vi "NavbalLabVIEW(15-5-21).vi"() -> ()   [LabVIEW 2010]
uses:
  <vilib>/Analysis/Matrix/Datatypes/RealMatrix.ctl
  <vilib>/Utility/NIReport.llb/HTML Report Image Alignment.ctl
  <vilib>/Utility/NIReport.llb/NI_report.lvclass
  <vilib>/Analysis/Matrix/Datatypes/ComplexMatrix.ctl
  <userlib>/Circular Buffer/Controls/Circular Buffer Operations.ctl
  <vilib>/addons/_office/_exclsub.llb/font.ctl
  <vilib>/addons/_office/excel.llb/Excel Get Data ([str]).vi
  <vilib>/addons/_office/excel.llb/Excel Get Data ([i32]).vi
  <vilib>/Analysis/Matrix/Numeric/Multiply/Multiply - R,RM.vi
  <vilib>/Analysis/Matrix/Numeric/Complex/Polar To Complex - RM,RM.vi
  <vilib>/Analysis/Matrix/Numeric/Conversions/Matrix To Array - RM.vi
  <vilib>/Analysis/Matrix/Numeric/Conversions/Array To Matrix - CA2.vi
  <vilib>/Analysis/Matrix/Numeric/Multiply/Multiply - RM,R.vi
  <vilib>/Analysis/baseanly.llb/Complex A x B.vi
  <vilib>/Analysis/Matrix/Numeric/Add/Add - CM,CM.vi
  <vilib>/Analysis/Matrix/Numeric/Complex/Complex To Polar - CM.vi
  <vilib>/Analysis/Matrix/Numeric/Subtract/Subtract - RM,RM.vi
  <vilib>/addons/_office/excel.llb/Excel Get Data ([dbl]).vi
  <userlib>/Circular Buffer/Instance VIs/Circular Buffer(2D Wfm with Attributes).vi
  <vilib>/addons/_office/excel.llb/Excel Easy Table (str).vi
  <vilib>/addons/_NISVFA/_Shared subVIs/Common/SVL Set dB Reference (N Ch - 1 Ref).vi
  <vilib>/measure/matone.llb/Extract Single Tone Information N Chan.vi
  <vilib>/Analysis/NI_AALPro.lvlib
  <vilib>/Utility/NIReport.llb/NI_ReportGenerationCore.lvlib
  <vilib>/Analysis/Matrix/NI_Matrix.lvlib
  <userlib>/Circular Buffer/Circular Buffer.lvlib
  <vilib>/measure/NI_MAPro.lvlib
  <vilib>/Utility/NIReport.llb/Excel/NI_Excel.lvclass
  <vilib>/addons/_office/NI_ReportGenerationToolkit.lvlib
  <vilib>/ptbypt/NI_PtbyPt.lvlib
  <vilib>/Analysis/NI_AALBase.lvlib
panel:
  in  "Print Button":bool caption="Blank Button"
  in  "Averaging":bool
  in  "Number of Averages":i32=100
  in  "Tab 2":T1(tab)
  in  "Save BG":bool
  out "XY Graph":cluster{"y vector":sgl[], dbl[]}[](graph)
  out "Port 60":dbl[](array[numeric])
  out "Stbd 60":dbl[](array[numeric])
  out "Corners 60":dbl[](array[numeric])
  out "Corners 120":dbl[](array[numeric])
  out "Stbd 120":dbl[](array[numeric])
  out "Port 120":dbl[](array[numeric])
  out "Sensor Name":string
  out "AdB Starboard":cluster{"x0":dbl, "dx":dbl, dbl[][]}(graph)={"x0"=0.0, "dx"=0.25, []}
  out "Accelerometer Signals Stbd":dynamicdata(graph) caption="Signal Out"
  out "Tach Signal Stbd":dynamicdata(graph) caption="Signal Out"
  out "AdB Port":cluster{"x0":dbl, "dx":dbl, dbl[][]}(graph)={"x0"=0.0, "dx"=0.25, []}
  out "Accelerometer Signals Port":dynamicdata(graph) caption="Signal Out"
  out "Tach Signal Port":dynamicdata(graph) caption="Signal Out"
  out "AdB Corners":cluster{"x0":dbl, "dx":dbl, dbl[][]}(graph)={"x0"=0.0, "dx"=0.25, []}
  out "Accelerometer Signals Corners":dynamicdata(graph) caption="Signal Out"
  in  "MagPhase":i32[](listbox)
  out "Spectrum (AdB)":cluster{"x0":dbl, "dx":dbl, dbl[][]}(graph)
  in  "Save Vibration Survey":bool
  in  "Vibration Survey Name":string
  out "Default Stbd Graph":dynamicdata(graph)
  in  "Enter into log":bool
  in  "Log Input":string
  out "Frequency (RPM) 1":i32=3573 caption="RPM"
  out "Frequency (Hz) 1":dbl=59.548178197923264 caption="Hz" format="%0.2f"
  out "Frequency (RPM) 2":i32=3621 caption="RPM"
  out "Frequency (Hz) 2":dbl=60.35080413674587 caption="Hz" format="%0.2f"
  in  "DAQ Start":bool
  in  "stop 4":bool
  in  "Tab 1":T2(tab)
  in  "Divisions in\nEach Plane S":T3=[[24.0], [24.0], [16.0], [16.0]]
  out "With/Against\nRotation S":string[][](array[string])
  in  "Load File":bool
  in  "Printer Name":string="HP LaserJet Professional P1102w"
  in  "Boat File":path
  in  "Frequency Resolution":u16(ring) items=["0.25 Hz", "0.5 Hz", "1 Hz", "5 Hz", "10 Hz"]
  in  "Frequency Upper Limit":u16(ring)=2 items=["200 Hz", "400 Hz", "800 Hz", "1600 Hz", "3200 Hz", "6400", "12.8 kHz"]
  in  "Ship Class":T4(radio)
  out "Number of Samples":i32
  out "Sample Frequency (Hz)":i32
  out "Sensor Info":string[][](array[string])
  out "sensor end line":cluster{"row":i32, i32}
  out "# Accel Channels":i32
  out "#Corner Accels":i32
  out "#Stbd Accels":i32
  out "#Port Accels":i32
  out "With/Against\nRotation P":string[][](array[string])
  in  "Divisions in\nEach Plane P":T3=[[24.0], [24.0], [16.0], [16.0]]
  in  "Calib Avg":bool
  in  "Accel Calib Start":bool
  out "mV/in/s":dbl
  out "Volts":dbl
  in  "Calibration Channel List":i32(listbox)
  out "FFT mV/in/s":cluster{"x0":dbl, "dx":dbl, "magnitude":dbl[]}[](graph)
  out "Volts Graph":dynamicdata(graph)=[{"t0"=timestamp(3478348950.00005 s since 1904-01-01), "dt"=4.999999999999997e-05, "Y"=array[10000 elements], "attributes"=variant("NI_ChannelName"=variant(string "Acceleration_10"), "NI_UnitDescription"=variant(string "g"), "NI_dBReference"=variant(dbl 1.0))}]
  in  "Save Calibration":bool
  in  "Corner Cluster Stbd":T5={"Amplitude"=5.0, "Phase"=5.0, "Amplitude 2"=5.0, "Phase 2"=5.0, "Amplitude 3"=7.0, "Phase 3"=55.0, "Amplitude 4"=5.0, "Phase 4"=55.0, "Amplitude 5"=5.0, "Phase 5"=55.0, "Amplitude 6"=5.0, "Phase 6"=55.0, "Amplitude 7"=5.0, "Phase 7"=55.0, "Amplitude 8"=5.0, "Phase 8"=55.0, "Amplitude 9"=5.0, "Phase 9"=55.0, "Amplitude 10"=5.0, "Phase 10"=55.0, "Amplitude 11"=5.0, "Phase 11"=55.0, "Amplitude 12"=5.0, "Phase 12"=55.0}
  in  "Stbd Cluster":T6={"Frequency"=59.5, "Amplitude"=5.0, "Amplitude 2"=0.0, "Amplitude 3"=0.0, "Amplitude 4"=0.0, "Amplitude 5"=0.0, "Amplitude 6"=0.0, "Amplitude 7"=0.0, "Amplitude 8"=0.0, "Amplitude 9"=0.0, "Phase"=32.0, "Phase 2"=0.0, "Phase 3"=0.0, "Phase 4"=0.0, "Phase 5"=0.0, "Phase 6"=0.0, "Phase 7"=0.0, "Phase 8"=0.0, "Phase 9"=0.0}
  in  "Port Cluster":T6={"Frequency"=60.5, "Amplitude"=10.0, "Amplitude 2"=0.0, "Amplitude 3"=0.0, "Amplitude 4"=0.0, "Amplitude 5"=0.0, "Amplitude 6"=0.0, "Amplitude 7"=0.0, "Amplitude 8"=0.0, "Amplitude 9"=0.0, "Phase"=39.0, "Phase 2"=0.0, "Phase 3"=0.0, "Phase 4"=0.0, "Phase 5"=0.0, "Phase 6"=0.0, "Phase 7"=0.0, "Phase 8"=0.0, "Phase 9"=0.0}
  in  "Corner Cluster Port":T5={"Amplitude"=5.0, "Phase"=12.0, "Amplitude 2"=5.0, "Phase 2"=12.0, "Amplitude 3"=4.0, "Phase 3"=90.0, "Amplitude 4"=5.0, "Phase 4"=12.0, "Amplitude 5"=5.0, "Phase 5"=12.0, "Amplitude 6"=5.0, "Phase 6"=12.0, "Amplitude 7"=5.0, "Phase 7"=12.0, "Amplitude 8"=5.0, "Phase 8"=12.0, "Amplitude 9"=5.0, "Phase 9"=12.0, "Amplitude 10"=5.0, "Phase 10"=12.0, "Amplitude 11"=5.0, "Phase 11"=12.0, "Amplitude 12"=5.0, "Phase 12"=12.0}
  in  "stop 2":bool
  in  "Tab 6":T7(tab)
  in  "phase data format":string(combo)="navbal"
  out "mag":dbl[](array[numeric])=[5.048747520166771, 5.048747520166771, 5.075144897278462, 5.078078052985233, 5.081196305358014, 5.096938449081231, 5.114146724243718, 5.128433984208956, 5.145287144412244, 5.16430129754644, 5.168163147560112]
  out "phase":dbl[](array[numeric])=[242.42996871547376, 242.42996871547376, 244.4144809819265, 242.62662099050746, 241.48608383332476, 244.21540251784086, 242.51619904336303, 241.29347697152338, 243.72328278239752, 243.1065553167647, 241.60880357150108]
  out "frequency resolution":dbl=0.25000000023283064
  out "Magnitude VdB Stbd":dbl[][](array[numeric])=[[74.92578260879114, 69.77256180693475, 59.3602001396654, 47.62612047007429, 50.77479123900201, 50.266598848862465, 47.770701022683625, 53.90683122328411], [82.5934638859237, 63.134491492071916, 56.32282870076566, 54.9658464020473, 49.954286595066876, 48.73501772409975, 46.78166981727508, 55.59661356931897], [79.12325810710927, 72.34721675639899, 51.87557402819359, 39.712634817643526, 49.33563866146112, 60.87557842567607, 45.392156674631146, 50.40568073521876], [16.06614035699032, 15.358272686755432, 16.336661959915112, 13.05753646153317, 16.008770873281193, 15.645215599158181, 15.495490367226942, 14.126952663655075], [17.87803484720246, 16.106114494426865, 16.62155539587407, 16.707041833791433, 16.442283946185373, 15.640084180883484, 15.816438726088824, 16.106851697052846], [16.842959089576958, 14.680333691029704, 15.729116811293835, 16.55864927252346, 15.111126179536807, 15.94032559227199, 17.059832115262747, 17.956593488913978], [16.758949506515396, 17.304836427787414, 15.242153558443587, 16.27870332888259, 15.072259512881272, 15.792072161686699, 17.28889122826976, 14.332760852594484], [16.301532847425342, 15.815993609067124, 14.40848526303014, 15.087256609638558, 15.39703005492566, 14.873689758385682, 15.580719211174944, 14.472767884888626], [16.94369202662193, 16.01328428880923, 15.726291225558764, 15.769308032358943, 14.966236460848027, 13.347849644037339, 15.0229573339147, 13.893160129623723], [17.289665346006906, 16.672193608742596, 16.41883394868716, 15.395715583117994, 15.672916989332254, 16.747708258755637, 15.82465755143936, 16.300674602559152], [16.98549849851792, 15.783415349358092, 16.820521090276696, 17.19524186827505, 14.873649562662463, 16.075731750857763, 15.53356465205735, 15.946319436410212], [27.80052546312017, 17.681235876365506, 18.46491074862667, 17.005201795612404, 17.374231774369107, 16.64285268927385, 18.456671624543592, 18.953385672297113]]
  out "Magnitude AdB Stbd":dbl[][](array[numeric])=[[66.39520970888674, 61.24198890703035, 50.829627239761, 39.09554757016989, 42.244218339097614, 41.736025948958066, 39.240128122779225, 45.37625832337971], [74.0628909860193, 54.60391859216752, 47.79225580086126, 46.4352735021429, 41.423713695162476, 40.20444482419535, 38.25109691737068, 47.06604066941457], [70.59268520720487, 63.81664385649459, 43.34500112828919, 31.182061917739126, 40.80506576155672, 52.34500552577167, 36.861583774726746, 41.87510783531436], [7.53556745708592, 6.827699786851031, 7.806089060010711, 4.526963561628769, 7.478197973376792, 7.11464269925378, 6.964917467322541, 5.596379763750674], [9.34746194729806, 7.5755415945224645, 8.090982495969667, 8.176468933887032, 7.911711046280972, 7.109511280979083, 7.285865826184423, 7.576278797148445], [8.312386189672557, 6.149760791125303, 7.198543911389434, 8.02807637261906, 6.580553279632406, 7.409752692367588, 8.529259215358346, 9.426020589009577], [8.228376606610995, 8.774263527883013, 6.7115806585391855, 7.748130428978188, 6.541686612976871, 7.261499261782298, 8.75831832836536, 5.802187952690083], [7.770959947520941, 7.285420709162723, 5.8779123631257395, 6.556683709734157, 6.8664571550212585, 6.343116858481281, 7.050146311270543, 5.942194984984225], [8.41311912671753, 7.48271138890483, 7.195718325654363, 7.238735132454542, 6.435663560943626, 4.817276744132938, 6.492384434010299, 5.362587229719322], [8.759092446102505, 8.141620708838195, 7.888261048782757, 6.865142683213593, 7.142344089427853, 8.217135358851236, 7.294084651534959, 7.770101702654751], [8.454925598613519, 7.252842449453691, 8.289948190372295, 8.66466896837065, 6.343076662758062, 7.545158850953362, 7.0029917521529494, 7.415746536505811], [19.269952563215767, 9.150662976461104, 9.93433784872227, 8.474628895708003, 8.843658874464706, 8.11227978936945, 9.926098724639191, 10.422812772392712]]
  out "Phase Stbd":dbl[][](array[numeric])=[[351.26804594724086, 268.6926717260623, 266.5059300328474, 218.19128619762265, 55.13201695417962, 288.47638623782086, 190.4242981093083, 51.58578084486782], [238.72076339767017, 262.415810828893, 140.91216410689412, 336.4741395508334, 272.3447618721675, 74.5759765524054, 6.042752248482757, 238.20554451194016], [241.39335546013197, 94.99844787872212, 348.08852683207715, 299.2855862425181, 349.7897961080541, 17.063494896214507, 100.02327184053524, 7.817529118469314], [252.09167903508722, 144.25468393857736, 40.184895103720116, 332.48301176715137, 181.58433762418048, 333.4842556226388, 281.8463821521221, 106.94808636615329], [52.61805580043213, 185.5893360617425, 171.08053334257346, 105.01013976081364, 223.91370704585228, 326.94671114070445, 10.736645011361459, 339.2843274933554], [262.50488768010507, 6.783647119235745, 2.0232854708041104, 283.77305001008483, 197.47093427743206, 44.35239098018768, 114.34223594970422, 95.41726761228514], [233.46766091275333, 109.78756294639757, 7.122663174520811, 115.55185636665152, 235.58090804380623, 123.33682322504411, 284.12352766631574, 0.42224140828222184], [182.55031689831827, 346.547526430712, 137.33887655610158, 309.28435686898246, 6.574599991125637, 228.53512044454615, 356.50309283760146, 203.85253908742095], [284.2803013767615, 85.24989147772851, 233.33707692954152, 18.703342054967145, 183.23121125820091, 305.5721997111382, 143.91573195842815, 31.47502028826888], [146.6563831237174, 191.71374112257357, 20.297552847044635, 284.69861665874333, 173.75867191415531, 122.55910913869288, 23.505947591477465, 110.85117567928442], [245.13717706847075, 228.1255626514732, 41.358212014605925, 147.38739616882933, 355.02301631709105, 276.7318219187853, 206.70609238248758, 302.67849438338254], [282.018187269307, 65.86279587559912, 304.6783319050354, 144.65838605091673, 137.40337794122624, 311.87147878628946, 340.181380512936, 66.46028142125459]]
  out "Freq Stbd":dbl[][](array[numeric])=[[59.548178197923264, 119.09635639584653, 178.64453459376978, 238.19271279169305, 297.74089098961633, 357.28906918753955, 416.83724738546283, 476.3854255833861], [59.548178197923264, 119.09635639584653, 178.64453459376978, 238.19271279169305, 297.74089098961633, 357.28906918753955, 416.83724738546283, 476.3854255833861], [59.548178197923264, 119.09635639584653, 178.64453459376978, 238.19271279169305, 297.74089098961633, 357.28906918753955, 416.83724738546283, 476.3854255833861], [59.548178197923264, 119.09635639584653, 178.64453459376978, 238.19271279169305, 297.74089098961633, 357.28906918753955, 416.83724738546283, 476.3854255833861], [59.548178197923264, 119.09635639584653, 178.64453459376978, 238.19271279169305, 297.74089098961633, 357.28906918753955, 416.83724738546283, 476.3854255833861], [59.548178197923264, 119.09635639584653, 178.64453459376978, 238.19271279169305, 297.74089098961633, 357.28906918753955, 416.83724738546283, 476.3854255833861], [59.548178197923264, 119.09635639584653, 178.64453459376978, 238.19271279169305, 297.74089098961633, 357.28906918753955, 416.83724738546283, 476.3854255833861], [59.548178197923264, 119.09635639584653, 178.64453459376978, 238.19271279169305, 297.74089098961633, 357.28906918753955, 416.83724738546283, 476.3854255833861], [59.548178197923264, 119.09635639584653, 178.64453459376978, 238.19271279169305, 297.74089098961633, 357.28906918753955, 416.83724738546283, 476.3854255833861], [59.548178197923264, 119.09635639584653, 178.64453459376978, 238.19271279169305, 297.74089098961633, 357.28906918753955, 416.83724738546283, 476.3854255833861], [59.548178197923264, 119.09635639584653, 178.64453459376978, 238.19271279169305, 297.74089098961633, 357.28906918753955, 416.83724738546283, 476.3854255833861], [59.548178197923264, 119.09635639584653, 178.64453459376978, 238.19271279169305, 297.74089098961633, 357.28906918753955, 416.83724738546283, 476.3854255833861]]
  out "Mils/sec Stbd":dbl[][](array[numeric])=[[3.11039557895813, 1.7185199804937212, 0.5182466488592785, 0.13422472381399145, 0.19287061151731716, 0.18190994307423886, 0.1364776534086121, 0.27661011465271335], [7.5196857177549195, 0.8002967811138507, 0.3653153580375145, 0.31247754623689156, 0.1754853334525778, 0.15250264695990068, 0.12178953894383557, 0.33601384631283615], [5.043005024575788, 2.311465061506275, 0.21892995960029013, 0.05397072305150428, 0.16342121256452316, 0.617028773668431, 0.10378493776733719, 0.18484620227159412], [0.0035467739771152798, 0.0032691897594709727, 0.0036589762750016473, 0.0025084376959821427, 0.003523425062326223, 0.003378992870750459, 0.003321245766783598, 0.002837096635275438], [0.004369464727658013, 0.0035631345325754815, 0.0037809790005061588, 0.003818375081628871, 0.0037037417134344014, 0.0033769972311839323, 0.0034462631146835823, 0.0035634369614247624], [0.0038785951494015244, 0.0030237311923648324, 0.0034117903467123897, 0.0037536948035066632, 0.0031774798451226567, 0.0034957693891204266, 0.003976656707248069, 0.004409163158706957], [0.003841262361277083, 0.004090423896504964, 0.003225775755088875, 0.0036346421774085366, 0.0031632933703938017, 0.003436608845524569, 0.004082921752456967, 0.002905123089848686], [0.003644207838075431, 0.0034460865120403577, 0.002930560952469206, 0.0031687598450503857, 0.0032838098275814356, 0.0030917970853276884, 0.003353995349290322, 0.0029523299329598123], [0.00392383825382197, 0.003525256401946162, 0.0034106806459593244, 0.0034276139139917737, 0.0031249157903707756, 0.0025936954353176257, 0.003145388989573912, 0.0027617508859076653], [0.004083285653350098, 0.0038030862594804803, 0.00369375590872156, 0.0032833129125823604, 0.003389786493917832, 0.0038362942286293855, 0.0034495256059931903, 0.003643847774997843], [0.0039427697914630865, 0.0034331854474913153, 0.0038685886207333064, 0.004039137046927427, 0.003091782777440126, 0.0035506926655830386, 0.0033358362832892636, 0.003498182536065246], [0.01369470774934442, 0.004271577490912595, 0.004674896852018887, 0.00395172382455052, 0.004123234966837133, 0.003790261114835882, 0.004670464514668517, 0.004945335715382192]]
  out "Mils(1x) Stbd":dbl[](array[numeric])=[0.016591568771143303, 0.04011174127417775, 0.026900554143179843, 1.8919311985622442e-05, 2.3307734557128735e-05, 2.0689322796129295e-05, 2.0490181077379598e-05, 1.9439046715087258e-05, 2.0930659969924818e-05, 2.1781189244254945e-05, 2.103164516641911e-05, 7.305073572026695e-05]
  out "Starboard Arrays":dbl[][](array[numeric])
  out "Phase Port":dbl[][](array[numeric])=[[268.11311412057194, 103.64053733275506, 178.1748723975787, 179.28661895777088, 272.7916850051796, 355.4145710762009, 172.14035422296925, 170.62439621635565], [173.37394203645292, 281.65738403333256, 299.288657788572, 131.78158177247403, 157.32393425255597, 102.44636485054096, 24.80814114080235, 95.45580821402676], [271.8991934006091, 157.35143822148206, 2.7542507044129736, 341.76736103459115, 258.71342396984153, 315.8460516245828, 206.56738579717396, 267.2328650367116], [34.25758619942892, 277.1399336728177, 164.41504387181632, 47.816487694039665, 266.6621943152023, 349.7888967081687, 273.4421428853626, 203.80985039109333], [216.8523700664608, 65.27907166452877, 86.07099446289263, 56.73652276282569, 298.836123181489, 96.00864814213473, 105.6015289981739, 150.31515595950648], [78.78163716645659, 40.319879842321086, 79.10495149694667, 341.129810708013, 315.35059786816896, 226.1690329050137, 341.3580396853242, 100.1110011836267], [24.50622346477741, 36.533321147485466, 295.5632097011204, 94.23748930878207, 163.6276029666236, 10.766169998964347, 264.74642454493204, 120.8394910491875], [103.26138286209218, 204.12160594707862, 340.5927346019335, 91.23101965058967, 297.3242782182021, 81.95293773650384, 250.90187096137333, 154.1808951870655], [140.86984174771032, 52.993657211153725, 319.60405993911075, 40.99568501671829, 139.89429510276636, 9.625663419477604, 314.20570701208646, 304.14738192862836], [77.47717355912859, 0.7120260000105386, 28.92922663289231, 357.93871117594585, 118.8535039435165, 192.95018194127692, 51.76989459334084, 59.31958735354357], [303.0257961882641, 276.4388139454717, 256.20444914445494, 11.400638851235346, 290.90312400978416, 33.54453964429952, 93.1672943557808, 39.58187201827054], [286.98189201997275, 279.48656604365254, 62.012616211324335, 342.72969735517626, 198.2027332764226, 196.31640901162945, 54.83131480265282, 34.223360107091544]]
  out "Magnitude VdB Port":dbl[][](array[numeric])=[[63.49402678413004, 76.27966745201802, 42.53034170466074, 48.21534470676946, 44.93890816241943, 43.611613904144065, 48.84065215909943, 55.654509321328135], [66.0043654563491, 68.59131629610766, 53.69863126553479, 44.28098476225746, 54.97838891116878, 57.33457159680733, 51.97751151647046, 58.904935564465355], [70.27026481447402, 69.67621883130454, 56.08376659917535, 49.22367266021888, 62.96908610369557, 57.739149833643275, 57.44458364151821, 63.21723038077738], [17.424549384841633, 15.687850426258246, 16.037306138004052, 17.389706638342815, 15.79372787748321, 16.20303029508894, 18.458395298412306, 17.87831494330948], [18.23292542858479, 16.84609309196808, 18.290084157573876, 17.278577139400706, 17.609925727870483, 18.43744278679629, 19.264146749553927, 22.806440302413545], [16.84169207385661, 17.80511916863613, 17.594771742745543, 15.53014794637399, 16.78378451974415, 16.302009344983034, 18.734685976037497, 18.599761654560538], [15.375715795236042, 15.074312163583468, 17.053502311201754, 17.82819356432587, 17.026350810769074, 16.674120596883267, 15.419092108096887, 16.32495517896534], [17.10508495009433, 16.751657715820798, 15.342517048374019, 15.69909005178565, 16.997574972782427, 15.743940655828773, 16.493040102074595, 14.541547494577625], [14.25452885517686, 14.825799146315353, 16.055499009728674, 17.744368642486453, 13.962141678848322, 16.629335929976726, 15.811329001839221, 15.346960178730999], [16.45565800660165, 16.415767198293974, 13.712913169034959, 14.78650181054385, 16.052327781739898, 15.162935505302102, 14.48899915587945, 14.616563666630775], [16.48430998194671, 17.725181003443986, 16.515669985350694, 16.458890330787767, 17.27222198272932, 15.62084612931846, 14.76886938037821, 14.801454770270752], [15.700135457964917, 17.757482097260638, 15.536946939217714, 15.343170884628714, 15.68779677435866, 16.135854256029535, 16.715810047288088, 16.358210269463758]]
  out "Magnitude AdB Port":dbl[][](array[numeric])=[[55.07974552121017, 67.86538618909815, 34.11606044174087, 39.801063443849586, 36.52462689949956, 35.19733264122419, 40.426370896179556, 47.24022805840826], [57.590084193429234, 60.17703503318779, 45.28435000261492, 35.86670349933759, 46.56410764824891, 48.92029033388746, 43.563230253550586, 50.49065430154548], [61.85598355155415, 61.26193756838467, 47.66948533625548, 40.80939139729901, 54.554804840775695, 49.3248685707234, 49.030302378598336, 54.80294911785751], [9.01026812192176, 7.273569163338372, 7.6230248750841785, 8.975425375422942, 7.379446614563337, 7.788749032169067, 10.044114035492433, 9.464033680389607], [9.818644165664915, 8.431811829048206, 9.875802894654003, 8.864295876480833, 9.19564446495061, 10.023161523876416, 10.849865486634053, 14.392159039493672], [8.427410810936736, 9.390837905716255, 9.18049047982567, 7.115866683454117, 8.369503256824276, 7.887728082063161, 10.320404713117624, 10.185480391640665], [6.961434532316169, 6.660030900663594, 8.63922104828188, 9.413912301405995, 8.6120695478492, 8.259839333963393, 7.004810845177014, 7.910673916045466], [8.690803687174457, 8.337376452900925, 6.928235785454145, 7.284808788865776, 8.583293709862554, 7.3296593929089, 8.078758839154721, 6.127266231657751], [5.840247592256986, 6.411517883395479, 7.641217746808801, 9.33008737956658, 5.547860415928449, 8.215054667056853, 7.397047738919348, 6.932678915811126], [8.041376743681775, 8.0014859353741, 5.2986319061150855, 6.372220547623977, 7.638046518820024, 6.748654242382228, 6.074717892959576, 6.2022824037109014], [8.070028719026835, 9.310899740524112, 8.101388722430821, 8.044609067867894, 8.857940719809447, 7.206564866398587, 6.354588117458336, 6.387173507350878], [7.285854195045044, 9.343200834340765, 7.12266567629784, 6.928889621708841, 7.273515511438786, 7.721572993109662, 8.301528784368214, 7.943929006543884]]
  out "Mils/sec Port":dbl[][](array[numeric])=[[0.8341186558667776, 3.6350456406401443, 0.07465236670863186, 0.14364606410696043, 0.09850809116446227, 0.08454874990412917, 0.1543686490498299, 0.33826102581181616], [1.1136398632851499, 1.5000036309311768, 0.2700586291445206, 0.09132206716732011, 0.3129290927933471, 0.4104451000366966, 0.22151445490769664, 0.49178273027352776], [1.8198673616901961, 1.6995636624514592, 0.3553978739629287, 0.16132814066781212, 0.7852009216560454, 0.43001537830587044, 0.4156766961567066, 0.8079565657794006], [0.004147190306525557, 0.0033956194834815394, 0.003535019407218362, 0.004130587509387168, 0.0034372639988992674, 0.003603114059344281, 0.004671391438311897, 0.0043696056331777025], [0.004551690952214108, 0.003879994858607273, 0.0045817427719343174, 0.004078076350701193, 0.004236651897877438, 0.004660136468458511, 0.005125471618097013, 0.00770634611599018], [0.0038780294177577024, 0.004332937792309678, 0.004229266795213929, 0.0033345243475099064, 0.003852261155649974, 0.0036444077604596363, 0.0048223729471964395, 0.004748042287298568], [0.003275761582430183, 0.003164041008680549, 0.003973759791761469, 0.004344463708847137, 0.003961357483324039, 0.003803930078065511, 0.0032921612660619516, 0.0036540480543753254], [0.003997428854701247, 0.0038380389807650336, 0.0032632650372152734, 0.0034000162922060385, 0.003948255455680417, 0.003417618078148168, 0.0037254479549167618, 0.0029758008962748185], [0.002879074733892035, 0.003074797029449274, 0.0035424313772382094, 0.004302738253363807, 0.0027837714692124237, 0.0037843673944497392, 0.003444236347556334, 0.003264934736184854], [0.003709448926168785, 0.0036924519746031866, 0.002705030423370841, 0.0030609172300151604, 0.0035411382676659663, 0.003196489416078687, 0.0029578520925855607, 0.0030016128701219466], [0.0037217054172616775, 0.004293243743326985, 0.0037351667489291984, 0.003710829599103143, 0.004075093658505889, 0.003369525923541007, 0.003054709844544389, 0.003066191208093864], [0.0034004255320301932, 0.004309239185330112, 0.003337135511547877, 0.003263510690957904, 0.0033955985091334295, 0.003575355317537753, 0.003822231593032411, 0.0036680648817260853]]
  out "Freq Port":dbl[][](array[numeric])=[[60.35080413674587, 120.70160827349174, 181.05241241023762, 241.4032165469835, 301.7540206837294, 362.10482482047524, 422.4556289572211, 482.806433093967], [60.35080413674587, 120.70160827349174, 181.05241241023762, 241.4032165469835, 301.7540206837294, 362.10482482047524, 422.4556289572211, 482.806433093967], [60.35080413674587, 120.70160827349174, 181.05241241023762, 241.4032165469835, 301.7540206837294, 362.10482482047524, 422.4556289572211, 482.806433093967], [60.35080413674587, 120.70160827349174, 181.05241241023762, 241.4032165469835, 301.7540206837294, 362.10482482047524, 422.4556289572211, 482.806433093967], [60.35080413674587, 120.70160827349174, 181.05241241023762, 241.4032165469835, 301.7540206837294, 362.10482482047524, 422.4556289572211, 482.806433093967], [60.35080413674587, 120.70160827349174, 181.05241241023762, 241.4032165469835, 301.7540206837294, 362.10482482047524, 422.4556289572211, 482.806433093967], [60.35080413674587, 120.70160827349174, 181.05241241023762, 241.4032165469835, 301.7540206837294, 362.10482482047524, 422.4556289572211, 482.806433093967], [60.35080413674587, 120.70160827349174, 181.05241241023762, 241.4032165469835, 301.7540206837294, 362.10482482047524, 422.4556289572211, 482.806433093967], [60.35080413674587, 120.70160827349174, 181.05241241023762, 241.4032165469835, 301.7540206837294, 362.10482482047524, 422.4556289572211, 482.806433093967], [60.35080413674587, 120.70160827349174, 181.05241241023762, 241.4032165469835, 301.7540206837294, 362.10482482047524, 422.4556289572211, 482.806433093967], [60.35080413674587, 120.70160827349174, 181.05241241023762, 241.4032165469835, 301.7540206837294, 362.10482482047524, 422.4556289572211, 482.806433093967], [60.35080413674587, 120.70160827349174, 181.05241241023762, 241.4032165469835, 301.7540206837294, 362.10482482047524, 422.4556289572211, 482.806433093967]]
  out "Mils(1x) Port":dbl[](array[numeric])=[0.004390207814244756, 0.005861408800368322, 0.009578488451237033, 2.1827862454351537e-05, 2.395686638332319e-05, 2.0411190822748046e-05, 1.7241280956416687e-05, 2.1039624604199992e-05, 1.5153403302546712e-05, 1.9523902921563522e-05, 1.9588412380251176e-05, 1.789742339111604e-05]
  out "Port Arrays":dbl[][](array[numeric])
  out "Mils(1x) Corners":dbl[](array[numeric])=[0.0016463075843755977, 1.8969305612951837e-05, 5.983723158028009e-05, 0.002558124481620776, 0.0029396646492951452, 0.003007321203354988, 2.40443656093375e-05, 0.0029336486427493104, 2.3805543379285445e-05, 0.003238896134282664, 0.0031424857560161203, 0.0027674206890101853]
  out "Freq Corner":dbl[][](array[numeric])=[[60.35080413674587, 120.70160827349174, 181.05241241023762, 241.4032165469835, 301.7540206837294, 362.10482482047524, 422.4556289572211, 482.806433093967], [60.35080413674587, 120.70160827349174, 181.05241241023762, 241.4032165469835, 301.7540206837294, 362.10482482047524, 422.4556289572211, 482.806433093967], [60.35080413674587, 120.70160827349174, 181.05241241023762, 241.4032165469835, 301.7540206837294, 362.10482482047524, 422.4556289572211, 482.806433093967], [60.35080413674587, 120.70160827349174, 181.05241241023762, 241.4032165469835, 301.7540206837294, 362.10482482047524, 422.4556289572211, 482.806433093967], [60.35080413674587, 120.70160827349174, 181.05241241023762, 241.4032165469835, 301.7540206837294, 362.10482482047524, 422.4556289572211, 482.806433093967], [60.35080413674587, 120.70160827349174, 181.05241241023762, 241.4032165469835, 301.7540206837294, 362.10482482047524, 422.4556289572211, 482.806433093967], [60.35080413674587, 120.70160827349174, 181.05241241023762, 241.4032165469835, 301.7540206837294, 362.10482482047524, 422.4556289572211, 482.806433093967], [60.35080413674587, 120.70160827349174, 181.05241241023762, 241.4032165469835, 301.7540206837294, 362.10482482047524, 422.4556289572211, 482.806433093967], [60.35080413674587, 120.70160827349174, 181.05241241023762, 241.4032165469835, 301.7540206837294, 362.10482482047524, 422.4556289572211, 482.806433093967], [60.35080413674587, 120.70160827349174, 181.05241241023762, 241.4032165469835, 301.7540206837294, 362.10482482047524, 422.4556289572211, 482.806433093967], [60.35080413674587, 120.70160827349174, 181.05241241023762, 241.4032165469835, 301.7540206837294, 362.10482482047524, 422.4556289572211, 482.806433093967], [60.35080413674587, 120.70160827349174, 181.05241241023762, 241.4032165469835, 301.7540206837294, 362.10482482047524, 422.4556289572211, 482.806433093967]]
  out "Mils/sec Corner":dbl[][](array[numeric])=[[0.31279063031299537, 0.00500988422090608, 0.004068227022098284, 0.0040300688280997445, 0.0029636446448533843, 0.0033533417348935277, 0.0031918283990501313, 0.002638741182515112], [0.003604078068756174, 0.003577894140733259, 0.0041265667573608545, 0.0035066582851210073, 0.0032821547143865805, 0.003146905371609203, 0.0027095233282579036, 0.003563764931609947], [0.011368790109339855, 0.005496680145839973, 0.005052531582642785, 0.0031944684152000326, 0.003237506476635729, 0.003340045388666653, 0.0038112193678440836, 0.0033024745196781067], [0.4860315147784163, 0.008237252784182005, 0.05431840365860553, 0.010139755015148164, 0.011325351961560332, 0.015523374543997858, 0.026431288187998347, 0.003604390701450413], [0.5585223364627829, 0.006510095400957736, 0.06334759624142879, 0.010795726554468732, 0.012396207768768912, 0.01639754386640331, 0.03134360821654077, 0.005550568016296178], [0.5713767607453569, 0.00508621545978539, 0.06394485953466685, 0.011474292196915509, 0.013067530133244598, 0.01630015453329888, 0.031853013546037666, 0.003930425096659083], [0.004568315390026738, 0.0046898244658337045, 0.004045783409189813, 0.002922277268013181, 0.004442810460870202, 0.004359133019129764, 0.003774296679528068, 0.0040341556749539575], [0.5573793237613306, 0.007117783328889763, 0.062370147700758584, 0.012374617858466419, 0.01203184192186513, 0.01606927760992575, 0.03018844559404105, 0.004256320044164225], [0.004522940299381651, 0.0029660083804497204, 0.0038637740718335586, 0.0037058570692827617, 0.0038822753814702284, 0.004159249059425955, 0.0034424600317106303, 0.0037798046118679516], [0.6153748989407957, 0.01694605801796116, 0.06250193646860305, 0.010593413276289942, 0.013643585631323632, 0.014852694420296525, 0.030200912639841017, 0.004309778703023988], [0.5970573844781843, 0.013675957940529001, 0.06243576632733528, 0.012288497141949274, 0.013619676249351198, 0.016812587420753214, 0.03020010850624203, 0.0041125736304141475], [0.5257968012004444, 0.00877391214422234, 0.055611940161385195, 0.00845280371885997, 0.010319005405287095, 0.01412379026708107, 0.02736114274688182, 0.0048790957771036175]]
  out "Magnitude AdB Corner":dbl[][](array[numeric])=[[46.560263531470845, 10.651742614448567, 8.843292430126075, 8.76143809413668, 6.09171139578519, 7.164745108768065, 6.735979517089373, 5.083124728885197], [7.791072622067292, 7.72773856559286, 8.966966332514295, 7.553057767998029, 6.978369806782327, 6.612862501732687, 5.313046717288893, 7.693369825781433], [17.769473799068244, 11.457198145255004, 10.72536956500865, 6.7431607962857285, 6.859401744791185, 7.130236198496286, 8.276467762950487, 7.031978336653236], [50.38847743229084, 14.970836702533743, 31.35412878998909, 16.77573807107199, 17.736222978897814, 20.474911550004272, 25.09755542608061, 7.791826039517703], [51.59599974951497, 12.926935884872636, 32.689791626748345, 17.320226341970468, 18.52096576076434, 20.950764854697013, 26.578168630152533, 11.541937403615654], [51.79364027914022, 10.783083898874116, 32.771301580955914, 17.84970692985602, 18.97905903161601, 20.89902326173236, 26.718199352748805, 8.543979310949863], [9.850310413834494, 10.078320585435817, 8.795241409334272, 5.969617222101297, 9.608344542250356, 9.443191261544696, 8.191909526781073, 8.770241892634344], [51.57820591336304, 13.702084098694522, 32.55472427723704, 18.505824753476887, 18.26183117459741, 20.775115899054, 26.25200386153982, 9.235874352579016], [9.763605932999043, 6.098636302697358, 8.395423302714297, 8.032962128029537, 8.43691558603218, 9.035487368299888, 7.392566959488809, 8.20457583851577], [52.437984376041186, 21.236562606071097, 32.57305828880828, 17.15590713800802, 19.353759246835438, 20.09129374600696, 26.255590168420262, 9.344288241563634], [52.17551030922565, 19.374343956528783, 32.56385775789944, 18.4451642830088, 19.33852451026749, 21.167879938098963, 26.25535889366487, 8.93746255724348], [51.07154761991759, 15.519054454286335, 31.558549762625795, 15.195204515120222, 16.92794562575711, 19.654214023472683, 25.39787346435203, 10.421975695594439]]
  out "Magnitude VdB Corner":dbl[][](array[numeric])=[[54.97454479439072, 19.06602387736844, 17.25757369304595, 17.175719357056554, 14.505992658705063, 15.579026371687938, 15.150260780009246, 13.49740599180507], [16.205353884987165, 16.142019828512733, 17.381247595434168, 15.967339030917902, 15.3926510697022, 15.02714376465256, 13.727327980208766, 16.107651088701306], [26.183755061988116, 19.871479408174878, 19.139650827928524, 15.157442059205602, 15.273683007711059, 15.54451746141616, 16.69074902587036, 15.446259599573109], [58.80275869521071, 23.385117965453617, 39.76841005290896, 25.190019333991863, 26.15050424181769, 28.889192812924144, 33.51183668900048, 16.206107302437577], [60.01028101243484, 21.34121714779251, 41.10407288966822, 25.73450760489034, 26.935247023684212, 29.365046117616885, 34.992449893072404, 19.956218666535527], [60.20792154206009, 19.19736516179399, 41.185582843875785, 26.263988192775894, 27.393340294535882, 29.313304524652235, 35.132480615668676, 16.958260573869737], [18.264591676754367, 18.49260184835569, 17.209522672254145, 14.38389848502117, 18.02262580517023, 17.85747252446457, 16.606190789700946, 17.184523155554217], [59.992487176282914, 22.116365361614395, 40.969005540156914, 26.920106016396762, 26.676112437517286, 29.189397161973876, 34.66628512445969, 17.65015561549889], [18.177887195918917, 14.512917565617231, 16.80970456563417, 16.44724339094941, 16.851196848952053, 17.44976863121976, 15.806848222408682, 16.618857101435644], [60.85226563896106, 29.65084386899097, 40.98733955172815, 25.57018840092789, 27.76804050975531, 28.505575008926836, 34.669871431340134, 17.758569504483507], [60.58979157214552, 27.788625219448658, 40.97813902081931, 26.859445545928672, 27.75280577318736, 29.582161201018835, 34.66964015658474, 17.351743820163353], [59.48582888283746, 23.93333571720621, 39.972831025545666, 23.609485778040096, 25.342226888676983, 28.068495286392555, 33.8121547272719, 18.836256958514312]]
  out "frequency (resolution) corner":dbl=0.25000000023283064
  out "Phase Corner":dbl[][](array[numeric])=[[90.49045518989102, 239.79379492125662, 245.65190204324125, 36.881937109145404, 44.582886119948284, 169.8636052564232, 20.26559084051402, 200.1282096599407], [280.13726230226285, 348.10665275106936, 244.7657229984299, 281.49580576490814, 149.0504352521256, 340.36376088164633, 309.6453547186082, 355.7265794449492], [189.70166244221923, 208.29720700637867, 25.265613968297366, 74.15662078841811, 338.0278942215902, 333.91170242281123, 354.3019475552347, 22.384202620213234], [242.2603813657085, 144.60164486814608, 214.85485431025816, 87.84888472731203, 10.381613290672759, 163.16666286727482, 183.96317356719095, 5.493563458169352], [244.3186672545434, 19.103559603426607, 226.48471786604904, 110.7609267111955, 300.04411944196175, 183.5616601711432, 194.8945898556949, 297.7929881683626], [239.03946332474345, 116.19439718832126, 215.45705572142202, 193.38837619221331, 328.07612595333643, 145.87366314531212, 166.00105244946798, 262.86233563662546], [241.61576615620106, 237.7977621213882, 226.90477452395152, 229.64762677380125, 4.979163914440495, 355.1895895646222, 290.3642573753093, 340.03381614317306], [247.4690947548408, 103.37016152997533, 228.07100225835953, 171.2277508060861, 337.8943167572564, 115.46156764765776, 169.81121193079156, 298.0784309053853], [63.255975162202944, 38.77027370570779, 225.92627861166622, 284.22369262345046, 36.655754380237276, 266.393152137431, 234.84087095995824, 287.751714871511], [260.2578603872289, 115.57086517184158, 230.4814564755596, 111.6111011191152, 325.5811283046597, 177.01699835729104, 163.29298281497026, 151.5522035497891], [256.97420674986705, 65.16350166310296, 226.0927571393607, 37.21275900014844, 39.770047949354606, 144.20572491460658, 184.54241746535632, 24.61278664859549], [250.8379498721526, 1.3861744281600674, 228.73176703091022, 268.80948016906336, 243.56943455368176, 74.59559349741384, 165.50662166486617, 53.98837542248082]]
  out "Corner Arrays Stbd":dbl[][](array[numeric])
  out "Phase Corner 2":dbl[][](array[numeric])=[[90.49045518989102, 239.79379492125662, 245.65190204324125, 36.881937109145404, 44.582886119948284, 169.8636052564232, 20.26559084051402, 200.1282096599407], [280.13726230226285, 348.10665275106936, 244.7657229984299, 281.49580576490814, 149.0504352521256, 340.36376088164633, 309.6453547186082, 355.7265794449492], [189.70166244221923, 208.29720700637867, 25.265613968297366, 74.15662078841811, 338.0278942215902, 333.91170242281123, 354.3019475552347, 22.384202620213234], [242.2603813657085, 144.60164486814608, 214.85485431025816, 87.84888472731203, 10.381613290672759, 163.16666286727482, 183.96317356719095, 5.493563458169352], [244.3186672545434, 19.103559603426607, 226.48471786604904, 110.7609267111955, 300.04411944196175, 183.5616601711432, 194.8945898556949, 297.7929881683626], [239.03946332474345, 116.19439718832126, 215.45705572142202, 193.38837619221331, 328.07612595333643, 145.87366314531212, 166.00105244946798, 262.86233563662546], [241.61576615620106, 237.7977621213882, 226.90477452395152, 229.64762677380125, 4.979163914440495, 355.1895895646222, 290.3642573753093, 340.03381614317306], [247.4690947548408, 103.37016152997533, 228.07100225835953, 171.2277508060861, 337.8943167572564, 115.46156764765776, 169.81121193079156, 298.0784309053853], [63.255975162202944, 38.77027370570779, 225.92627861166622, 284.22369262345046, 36.655754380237276, 266.393152137431, 234.84087095995824, 287.751714871511], [260.2578603872289, 115.57086517184158, 230.4814564755596, 111.6111011191152, 325.5811283046597, 177.01699835729104, 163.29298281497026, 151.5522035497891], [256.97420674986705, 65.16350166310296, 226.0927571393607, 37.21275900014844, 39.770047949354606, 144.20572491460658, 184.54241746535632, 24.61278664859549], [250.8379498721526, 1.3861744281600674, 228.73176703091022, 268.80948016906336, 243.56943455368176, 74.59559349741384, 165.50662166486617, 53.98837542248082]]
  out "frequency (resolution) corners-port":dbl=0.25000000023283064
  out "Magnitude VdB Corners-Port":dbl[][](array[numeric])=[[54.97454479439072, 19.06602387736844, 17.25757369304595, 17.175719357056554, 14.505992658705063, 15.579026371687938, 15.150260780009246, 13.49740599180507], [16.205353884987165, 16.142019828512733, 17.381247595434168, 15.967339030917902, 15.3926510697022, 15.02714376465256, 13.727327980208766, 16.107651088701306], [26.183755061988116, 19.871479408174878, 19.139650827928524, 15.157442059205602, 15.273683007711059, 15.54451746141616, 16.69074902587036, 15.446259599573109], [58.80275869521071, 23.385117965453617, 39.76841005290896, 25.190019333991863, 26.15050424181769, 28.889192812924144, 33.51183668900048, 16.206107302437577], [60.01028101243484, 21.34121714779251, 41.10407288966822, 25.73450760489034, 26.935247023684212, 29.365046117616885, 34.992449893072404, 19.956218666535527], [60.20792154206009, 19.19736516179399, 41.185582843875785, 26.263988192775894, 27.393340294535882, 29.313304524652235, 35.132480615668676, 16.958260573869737], [18.264591676754367, 18.49260184835569, 17.209522672254145, 14.38389848502117, 18.02262580517023, 17.85747252446457, 16.606190789700946, 17.184523155554217], [59.992487176282914, 22.116365361614395, 40.969005540156914, 26.920106016396762, 26.676112437517286, 29.189397161973876, 34.66628512445969, 17.65015561549889], [18.177887195918917, 14.512917565617231, 16.80970456563417, 16.44724339094941, 16.851196848952053, 17.44976863121976, 15.806848222408682, 16.618857101435644], [60.85226563896106, 29.65084386899097, 40.98733955172815, 25.57018840092789, 27.76804050975531, 28.505575008926836, 34.669871431340134, 17.758569504483507], [60.58979157214552, 27.788625219448658, 40.97813902081931, 26.859445545928672, 27.75280577318736, 29.582161201018835, 34.66964015658474, 17.351743820163353], [59.48582888283746, 23.93333571720621, 39.972831025545666, 23.609485778040096, 25.342226888676983, 28.068495286392555, 33.8121547272719, 18.836256958514312]]
  out "Magnitude AdB Corners-Port":dbl[][](array[numeric])=[[46.560263531470845, 10.651742614448567, 8.843292430126075, 8.76143809413668, 6.09171139578519, 7.164745108768065, 6.735979517089373, 5.083124728885197], [7.791072622067292, 7.72773856559286, 8.966966332514295, 7.553057767998029, 6.978369806782327, 6.612862501732687, 5.313046717288893, 7.693369825781433], [17.769473799068244, 11.457198145255004, 10.72536956500865, 6.7431607962857285, 6.859401744791185, 7.130236198496286, 8.276467762950487, 7.031978336653236], [50.38847743229084, 14.970836702533743, 31.35412878998909, 16.77573807107199, 17.736222978897814, 20.474911550004272, 25.09755542608061, 7.791826039517703], [51.59599974951497, 12.926935884872636, 32.689791626748345, 17.320226341970468, 18.52096576076434, 20.950764854697013, 26.578168630152533, 11.541937403615654], [51.79364027914022, 10.783083898874116, 32.771301580955914, 17.84970692985602, 18.97905903161601, 20.89902326173236, 26.718199352748805, 8.543979310949863], [9.850310413834494, 10.078320585435817, 8.795241409334272, 5.969617222101297, 9.608344542250356, 9.443191261544696, 8.191909526781073, 8.770241892634344], [51.57820591336304, 13.702084098694522, 32.55472427723704, 18.505824753476887, 18.26183117459741, 20.775115899054, 26.25200386153982, 9.235874352579016], [9.763605932999043, 6.098636302697358, 8.395423302714297, 8.032962128029537, 8.43691558603218, 9.035487368299888, 7.392566959488809, 8.20457583851577], [52.437984376041186, 21.236562606071097, 32.57305828880828, 17.15590713800802, 19.353759246835438, 20.09129374600696, 26.255590168420262, 9.344288241563634], [52.17551030922565, 19.374343956528783, 32.56385775789944, 18.4451642830088, 19.33852451026749, 21.167879938098963, 26.25535889366487, 8.93746255724348], [51.07154761991759, 15.519054454286335, 31.558549762625795, 15.195204515120222, 16.92794562575711, 19.654214023472683, 25.39787346435203, 10.421975695594439]]
  out "Mils/sec Corners-Port":dbl[][](array[numeric])=[[0.31279063031299537, 0.00500988422090608, 0.004068227022098284, 0.0040300688280997445, 0.0029636446448533843, 0.0033533417348935277, 0.0031918283990501313, 0.002638741182515112], [0.003604078068756174, 0.003577894140733259, 0.0041265667573608545, 0.0035066582851210073, 0.0032821547143865805, 0.003146905371609203, 0.0027095233282579036, 0.003563764931609947], [0.011368790109339855, 0.005496680145839973, 0.005052531582642785, 0.0031944684152000326, 0.003237506476635729, 0.003340045388666653, 0.0038112193678440836, 0.0033024745196781067], [0.4860315147784163, 0.008237252784182005, 0.05431840365860553, 0.010139755015148164, 0.011325351961560332, 0.015523374543997858, 0.026431288187998347, 0.003604390701450413], [0.5585223364627829, 0.006510095400957736, 0.06334759624142879, 0.010795726554468732, 0.012396207768768912, 0.01639754386640331, 0.03134360821654077, 0.005550568016296178], [0.5713767607453569, 0.00508621545978539, 0.06394485953466685, 0.011474292196915509, 0.013067530133244598, 0.01630015453329888, 0.031853013546037666, 0.003930425096659083], [0.004568315390026738, 0.0046898244658337045, 0.004045783409189813, 0.002922277268013181, 0.004442810460870202, 0.004359133019129764, 0.003774296679528068, 0.0040341556749539575], [0.5573793237613306, 0.007117783328889763, 0.062370147700758584, 0.012374617858466419, 0.01203184192186513, 0.01606927760992575, 0.03018844559404105, 0.004256320044164225], [0.004522940299381651, 0.0029660083804497204, 0.0038637740718335586, 0.0037058570692827617, 0.0038822753814702284, 0.004159249059425955, 0.0034424600317106303, 0.0037798046118679516], [0.6153748989407957, 0.01694605801796116, 0.06250193646860305, 0.010593413276289942, 0.013643585631323632, 0.014852694420296525, 0.030200912639841017, 0.004309778703023988], [0.5970573844781843, 0.013675957940529001, 0.06243576632733528, 0.012288497141949274, 0.013619676249351198, 0.016812587420753214, 0.03020010850624203, 0.0041125736304141475], [0.5257968012004444, 0.00877391214422234, 0.055611940161385195, 0.00845280371885997, 0.010319005405287095, 0.01412379026708107, 0.02736114274688182, 0.0048790957771036175]]
  out "Freq Corner Port":dbl[][](array[numeric])=[[60.35080413674587, 120.70160827349174, 181.05241241023762, 241.4032165469835, 301.7540206837294, 362.10482482047524, 422.4556289572211, 482.806433093967], [60.35080413674587, 120.70160827349174, 181.05241241023762, 241.4032165469835, 301.7540206837294, 362.10482482047524, 422.4556289572211, 482.806433093967], [60.35080413674587, 120.70160827349174, 181.05241241023762, 241.4032165469835, 301.7540206837294, 362.10482482047524, 422.4556289572211, 482.806433093967], [60.35080413674587, 120.70160827349174, 181.05241241023762, 241.4032165469835, 301.7540206837294, 362.10482482047524, 422.4556289572211, 482.806433093967], [60.35080413674587, 120.70160827349174, 181.05241241023762, 241.4032165469835, 301.7540206837294, 362.10482482047524, 422.4556289572211, 482.806433093967], [60.35080413674587, 120.70160827349174, 181.05241241023762, 241.4032165469835, 301.7540206837294, 362.10482482047524, 422.4556289572211, 482.806433093967], [60.35080413674587, 120.70160827349174, 181.05241241023762, 241.4032165469835, 301.7540206837294, 362.10482482047524, 422.4556289572211, 482.806433093967], [60.35080413674587, 120.70160827349174, 181.05241241023762, 241.4032165469835, 301.7540206837294, 362.10482482047524, 422.4556289572211, 482.806433093967], [60.35080413674587, 120.70160827349174, 181.05241241023762, 241.4032165469835, 301.7540206837294, 362.10482482047524, 422.4556289572211, 482.806433093967], [60.35080413674587, 120.70160827349174, 181.05241241023762, 241.4032165469835, 301.7540206837294, 362.10482482047524, 422.4556289572211, 482.806433093967], [60.35080413674587, 120.70160827349174, 181.05241241023762, 241.4032165469835, 301.7540206837294, 362.10482482047524, 422.4556289572211, 482.806433093967], [60.35080413674587, 120.70160827349174, 181.05241241023762, 241.4032165469835, 301.7540206837294, 362.10482482047524, 422.4556289572211, 482.806433093967]]
  out "Mils(1x) Corners-Port":dbl[](array[numeric])=[0.0016463075843755977, 1.8969305612951837e-05, 5.983723158028009e-05, 0.002558124481620776, 0.0029396646492951452, 0.003007321203354988, 2.40443656093375e-05, 0.0029336486427493104, 2.3805543379285445e-05, 0.003238896134282664, 0.0031424857560161203, 0.0027674206890101853]
  out "Corner Arrays Port":dbl[][](array[numeric])
  out "Resid 0":dbl
  out "Final Mag 0":T3
  out "Final Phase 0":T3
  out "Final Phase 1":T3
  out "Resid 1":dbl
  out "Final Mag 1":T3
  out "Resid 2":dbl
  out "Final Mag  2":T3
  out "Final Phase 2":T3
  out "Final Mag 3":T3
  out "Final Phase 3":T3
  out "Resid 3":dbl
  out "Final Phase 4":T3
  out "Final Mag  5":T3
  out "Final Phase 5":T3
  out "Resid 5":dbl
  out "Final Mag  6":T3
  out "Final Phase 6":T3
  out "Resid 6":dbl
  out "Final Mag  7":T3
  out "Final Phase 7":T3
  out "Resid 7":dbl
  out "Resid 4":dbl
  out "Final Mag 4":T3
  out "Resid 8":dbl
  out "Final Mag 8":T3
  out "Final Phase 8":T3
  out "Resid 9":dbl
  out "Final Mag 9":T3
  out "Final Phase 9":T3
  out "Resid 10":dbl
  out "Final Mag 10":T3
  out "Final Phase 10":T3
  out "Final Phase 11":T3
  out "Final Mag 11":T3
  out "Resid 11":dbl
  out "Final Phase 12":T3
  out "Final Mag 12":T3
  out "Resid 12":dbl
  out "Final Phase 13":T3
  out "Final Mag 13":T3
  out "Resid 13":dbl
  out "Final Phase 14":T3
  out "Final Mag 14":T3
  out "Resid 14":dbl
  out "spectra":cluster{"x0":dbl, "dx":dbl, "magnitude":dbl[]}[](array[cluster])
  in  "Tab 5":T8(tab)
  in  "FG Reference":u16(ring) items=["Start Point", "Aft Turbine", "Fwd Turbine", "Aft Generator", "Ref A", "Ref B", "Ref C", "Ref D"]
  in  "AG Reference":u16(ring) items=["Start Point", "Aft Turbine", "Fwd Turbine", "Fwd Generator", "Ref A", "Ref B", "Ref C", "Ref D"]
  in  "FT Reference":u16(ring) items=["Start Point", "Aft Turbine", "Aft Generator", "Fwd Generator", "Ref A", "Ref B", "Ref C", "Ref D"]
  in  "AT Reference":u16(ring) items=["Start Point", "Fwd Turbine", "Aft Generator", "Fwd Generator", "Ref A", "Ref B", "Ref C", "Ref D"]
  in  "Empty Data Arrays":bool
  in  "Multicolumn Listbox":i32(listbox)
  in  "Base Select":bool
  in  "AT Select":bool
  out "Base Run":sgl[][](array[numeric])
  in  "FG Select":bool
  in  "AG Select":bool
  in  "FT Select":bool
  out "Base Wt":sgl[][](array[numeric])
  out "AT Wt":sgl[][](array[numeric])
  out "AT Run":sgl[][](array[numeric])
  out "FT Run":sgl[][](array[numeric])
  out "FT Wt":sgl[][](array[numeric])
  out "AG Run":sgl[][](array[numeric])
  out "AG Wt":sgl[][](array[numeric])
  out "FG Run":sgl[][](array[numeric])
  out "FG Wt":sgl[][](array[numeric])
  out "Base Available":bool
  out "1st Available":bool
  out "2nd Available":bool
  out "3rd Available":bool
  out "4th Available":bool
  in  "Select Side to Analyze":enum32{"Starboard", "Port"}(radio)
  in  "No. Runs":i32=15
  in  "Ref A Select":bool
  out "Ref A":cdb[][](array[numeric])
  in  "Ref B Select":bool
  out "Ref B":cdb[][](array[numeric])
  out "Ref C":cdb[][](array[numeric])
  in  "Refresh Button":bool
  in  "Ref C Select":bool
  out "Ref D":cdb[][](array[numeric])
  in  "Ref D Select":bool
  in  "Start Point:":u16(ring) items=["Stbd 2 BM (FT,AT)", "Stbd 2nd Eff (AT)", "Stbd 1 BM (FT)", "1st Effect - FT", "Base 3Peat", "", "", "", "", "", "", "", "", "", "", ""]
  out "Location":T3
  in  "Calc Response Coeff":bool
  out "Response Coefficients":cdb[][](array[numeric])
  in  "Iterative Solution?":bool
  in  "Calculate Solution":bool
  in  "Max Iteration Count":dbl=5.0
  in  "Solution Options":i32(listbox)
  in  "Ideal Weight":T3=[[0.0], [0.0], [0.0], [0.0]] format="%#.3g"
  in  "Avoid Occupancies":bool=TRUE
  in  "Omit AT":bool
  in  "Omit FT":bool
  in  "Omit AG":bool
  in  "Holes/Division":i32=10
  in  "Calculate 2 wt":bool
  in  "loc2":T3=[[0.0], [0.0], [0.0], [0.0]]
  in  "wt2":T3=[[0.0], [0.0], [0.0], [0.0]]
  in  "loc1":T3=[[0.0], [0.0], [0.0], [0.0]]
  in  "wt1":T3=[[0.0], [0.0], [0.0], [0.0]]
  in  "Split Weights":bool
  in  "Aft Turbine Balance Plane Split Options":i32(listbox)
  in  "Aft Generator Balance Plane Split Options":i32(listbox)
  in  "Fwd Generator Balance Plane Split Options":i32(listbox)
  in  "Fwd Turbine Balance Plane Split Options":i32(listbox)
  in  "Prediction Results":i32[](listbox)
  in  "Correction Mag":T3=[[0.0], [0.0], [0.0], [0.0]]
  in  "Weight Category AT":u16(ring) items=["1g increments", "0.5g increments", "Gen Reg", "Gen High Density", "Gen (ALL) Combined", "Turb Short", "Turb Long", "Turb (ALL) Combined", "Custom List", "", "", "", "", "", "", ""]
  in  "Weight Category FT":u16(ring) items=["1g increments", "0.5g increments", "Gen Reg", "Gen High Density", "Gen (ALL) Combined", "Turb Short", "Turb Long", "Turb (ALL) Combined", "Custom List", "", "", "", "", "", "", ""]
  in  "Weight Category AG":u16(ring) items=["1g increments", "0.5g increments", "Gen Reg", "Gen High Density", "Gen (ALL) Combined", "Turb Short", "Turb Long", "Turb (ALL) Combined", "Custom List", "", "", "", "", "", "", ""]
  in  "Weight Category FG":u16(ring) items=["1g increments", "0.5g increments", "Gen Reg", "Gen High Density", "Gen (ALL) Combined", "Turb Short", "Turb Long", "Turb (ALL) Combined", "Custom List", "", "", "", "", "", "", ""]
  in  "Correction Loc":T3=[[0.0], [0.0], [0.0], [0.0]]
  in  "Omit FG":bool
  in  "Existing Plane Wts Port":dbl[][](array[numeric])=[[0.0, 0.0, 18.4, 0.0], [0.0, 0.0, 0.0, 18.3], [0.0, 0.0, 18.2, 0.0], [0.0, 0.0, 18.4, 18.3], [0.0, 0.0, 0.0, 0.0], [0.0, 0.0, 0.0, 18.4], [0.0, 0.0, 18.4, 0.0], [0.0, 0.0, 0.0, 18.3], [0.0, 0.0, 18.4, 0.0], [0.0, 0.0, 18.4, 18.3], [0.0, 0.0, 0.0, 0.0], [0.0, 0.0, 51.5, 18.3], [0.0, 0.0, 50.0, 0.0], [0.0, 0.0, 0.0, 0.0], [0.0, 0.0, 18.4, 52.7], [0.0, 0.0, 0.0, 18.4], [0.0, 0.0, 18.2, 0.0], [0.0, 0.0, 0.0, 18.0], [0.0, 0.0, 0.0, 0.0], [0.0, 0.0, 18.3, 0.0], [0.0, 0.0, 0.0, 18.4], [0.0, 0.0, 18.4, 18.3], [0.0, 0.0, 18.4, 0.0], [0.0, 0.0, 0.0, 18.4], [0.0, 0.0, 18.3, 0.0], [0.0, 0.0, 0.0, 23.2], [0.0, 0.0, 18.3, 0.0], [0.0, 0.0, 0.0, 18.3], [0.0, 0.0, 18.2, 0.0], [0.0, 0.0, 0.0, 18.4], [0.0, 0.0, 18.4, 0.0], [0.0, 0.0, 0.0, 53.4], [0.0, 0.0, 0.0, 0.0], [0.0, 0.0, 0.0, 0.0], [0.0, 0.0, 0.0, 0.0], [0.0, 0.0, 0.0, 0.0], [0.0, 0.0, 0.0, 0.0], [0.0, 0.0, 0.0, 0.0], [0.0, 0.0, 0.0, 0.0], [0.0, 0.0, 0.0, 0.0], [0.0, 0.0, 0.0, 0.0], [0.0, 0.0, 0.0, 0.0], [0.0, 0.0, 0.0, 0.0], [0.0, 0.0, 0.0, 0.0], [0.0, 0.0, 0.0, 0.0], [0.0, 0.0, 0.0, 0.0], [0.0, 0.0, 0.0, 0.0], [0.0, 0.0, 0.0, 0.0]]
  out "Portloc":dbl[](array[numeric])
  in  "Solution Weighting Array":dbl[](array[numeric])=[1.0, 1.0, 1.0, 1.0, 1.0, 1.0, 1.0, 1.0, 1.0, 1.0, 1.0, 1.0, 1.0, 1.0, 1.0, 1.0, 1.0, 1.0, 1.0, 1.0, 1.0, 1.0, 1.0, 1.0, 1.0, 1.0, 1.0, 1.0, 1.0, 1.0, 1.0, 1.0, 1.0, 1.0, 1.0, 1.0]
  out "Sensor Column":string[](array[string])
  out "AT Weights":dbl[](array[numeric]) format="%.2f"
  out "FG Weights":dbl[](array[numeric]) format="%.2f"
  out "AG Weights":dbl[](array[numeric]) format="%.2f"
  out "FT Weights":dbl[](array[numeric]) format="%.2f"
  in  "Existing Plane Wts Stbd":dbl[][](array[numeric])=[[0.0, 0.0, 8.3, 10.5], [0.0, 0.0, 9.78, 0.0], [0.0, 0.0, 0.0, 18.1], [0.0, 0.0, 18.2, 0.0], [0.0, 0.0, 18.1, 20.8], [0.0, 0.0, 0.0, 0.0], [0.0, 0.0, 0.0, 18.1], [0.0, 0.0, 18.3, 0.0], [0.0, 0.0, 0.0, 10.7], [0.0, 0.0, 18.3, 0.0], [0.0, 0.0, 18.3, 31.2], [0.0, 0.0, 0.0, 0.0], [0.0, 0.0, 18.4, 18.3], [0.0, 0.0, 0.0, 0.0], [0.0, 0.0, 18.3, 42.2], [0.0, 0.0, 0.0, 18.3], [0.0, 0.0, 18.5, 0.0], [0.0, 0.0, 0.0, 19.4], [0.0, 0.0, 18.2, 0.0], [0.0, 0.0, 0.0, 0.0], [0.0, 0.0, 0.0, 47.9], [0.0, 0.0, 18.3, 0.0], [0.0, 0.0, 0.0, 52.5], [0.0, 0.0, 18.4, 0.0], [0.0, 0.0, 0.0, 0.0], [0.0, 0.0, 18.2, 18.0], [0.0, 0.0, 0.0, 0.0], [0.0, 0.0, 0.0, 18.3], [0.0, 0.0, 31.2, 18.4], [0.0, 0.0, 0.0, 0.0], [0.0, 0.0, 18.3, 10.8], [0.0, 0.0, 0.0, 0.0], [0.0, 0.0, 0.0, 0.0], [0.0, 0.0, 0.0, 0.0], [0.0, 0.0, 0.0, 0.0], [0.0, 0.0, 0.0, 0.0], [0.0, 0.0, 0.0, 0.0], [0.0, 0.0, 0.0, 0.0], [0.0, 0.0, 0.0, 0.0], [0.0, 0.0, 0.0, 0.0], [0.0, 0.0, 0.0, 0.0], [0.0, 0.0, 0.0, 0.0], [0.0, 0.0, 0.0, 0.0], [0.0, 0.0, 0.0, 0.0], [0.0, 0.0, 0.0, 0.0], [0.0, 0.0, 0.0, 0.0], [0.0, 0.0, 0.0, 0.0], [0.0, 0.0, 0.0, 0.0]]
  out "Solution Startpoint":sgl[][](array[numeric])
  out "Base Complex":cdb[][](array[numeric])
  out "Mils/Sec-Phase(CORNERS-Port)":sgl[][](array[numeric])=[[0.31279063, 90.490456], [0.003604078, 280.13727], [0.01136879, 189.70166], [0.4860315, 242.26038], [0.55852234, 244.31866], [0.57137674, 239.03946], [0.0045683156, 241.61577], [0.5573793, 247.4691], [0.00452294, 63.255974], [0.6153749, 260.25787], [0.5970574, 256.9742], [0.52579683, 250.83795]]
  out "Mils/Sec-Phase(CORNERS-Stbd)":sgl[][](array[numeric])=[[0.31279063, 90.490456], [0.003604078, 280.13727], [0.01136879, 189.70166], [0.4860315, 242.26038], [0.55852234, 244.31866], [0.57137674, 239.03946], [0.0045683156, 241.61577], [0.5573793, 247.4691], [0.00452294, 63.255974], [0.6153749, 260.25787], [0.5970574, 256.9742], [0.52579683, 250.83795]]
  out "Mils/Sec-Phase(STBD)":dbl[][](array[numeric])=[[3.11039557895813, 351.26804594724086], [7.5196857177549195, 238.72076339767017], [5.043005024575788, 241.39335546013197], [0.0035467739771152798, 252.09167903508722], [0.004369464727658013, 52.61805580043213], [0.0038785951494015244, 262.50488768010507], [0.003841262361277083, 233.46766091275333], [0.003644207838075431, 182.55031689831827], [0.00392383825382197, 284.2803013767615], [0.004083285653350098, 146.6563831237174], [0.0039427697914630865, 245.13717706847075], [0.01369470774934442, 282.018187269307]]
  out "Mils/Sec-Phase(PORT)":sgl[][](array[numeric])=[[0.83411866, 268.11313], [1.1136398, 173.37395], [1.8198674, 271.8992], [0.00414719, 34.257587], [0.004551691, 216.85237], [0.0038780295, 78.78164], [0.0032757616, 24.506224], [0.003997429, 103.26138], [0.0028790748, 140.86984], [0.003709449, 77.47717], [0.0037217054, 303.0258], [0.0034004254, 286.9819]]
  in  "Correction Phase":T3=[[0.0], [0.0], [0.0], [0.0]]
  in  "Degrees":T3=[[0.0], [0.0], [0.0], [0.0]]
  out "Startpt Complex":cdb[][](array[numeric])
  out "2wt-Exceptions":csg[](array[numeric])
  out "FG Exceptions":csg[](array[numeric])
  out "AG Exceptions":csg[](array[numeric])
  out "AT Exceptions":csg[](array[numeric])
  out "FT Exceptions":csg[](array[numeric])
  out "FT Complex":cdb[][](array[numeric])
  out "AG Complex":cdb[][](array[numeric])
  out "FG Complex":cdb[][](array[numeric])
  out "AT Complex":cdb[][](array[numeric])
  out "FG Correction 1":cdb
  out "FG Correction 2A":cdb
  out "FG Correction 2B":cdb
  out "AG Correction 1":cdb
  out "AG Correction 2B":cdb
  out "AG Correction 2A":cdb
  out "FT Correction 1":cdb
  out "FT Correction 2A":cdb
  out "FT Correction 2B":cdb
  out "AT Correction 1":cdb
  out "AT Correction 2A":cdb
  out "AT Correction 2B":cdb
  out "DataTab":i32
  out "Pred plot":dbl[][](array[numeric])
  out "With/Against\nRotation":string[][](array[string])
  in  "Divisions in\nEach Plane":T3=[[24.0], [24.0], [16.0], [16.0]]
  in  "Tab 4":enum32{"Dear Diary"}(tab)
  out "text":string="5:49:59 AM\nhere"
  out "Log File Path":string="C:\\Users\\Jim Gehringer\\Desktop\\Navbal-LabVIEW_FINAL\\balancelog.txt"
  in  "Tab 3":T9(tab)
  in  "# of Runs to include":i32=10
  in  "Clear Save array":bool
  in  "Automarker":bool
  in  "Marker Seconds":i32=100
  in  "Weight+Location":dbl[][](array[numeric])=[[0.0, 0.0, 0.0, 0.0], [0.0, 0.0, 0.0, 0.0], [0.0, 0.0, 0.0, 0.0], [0.0, 0.0, 0.0, 0.0]]
  in  "Save Run":bool
  out "Marker Time":string
  in  "Mark Current":bool
  out "Polar Plot Picture":picture
  in  "DAQ Listbox":i32(listbox)=2
  in  "Port/Starboard":enum32{"Port Side", "Stbd Side"}(radio)
  in  "Save Run As:":string
  in  "Run Reference:":u16(ring) items=["2BM-FT", "2E-FT", "1BM-AG", "1E-AG", "Base", "", "", "", "", ""]
  out "Indicate Ref":string
  in  "Clear Strtpt":bool
  in  "Slct Strt Pt":bool
  in  "Refresh Plot Listbox":bool
  in  "polar attributes Start Point":T10={"maximum"=0.0, "minimum"=0.0, "clip to min"=FALSE, "log?(F)"=FALSE, "grid color"=14145495, "plot color"=16711680, "fmt and prec"={"format"=enum."Decimal", "precision"=1}, "visible section"=8} {"minimum" format="%0.2f"; "maximum" format="%0.2f"}
  in  "polar attributes":T10={"maximum"=0.028203326380915113, "minimum"=0.0, "clip to min"=FALSE, "log?(F)"=FALSE, "grid color"=14145495, "plot color"=5892095, "fmt and prec"={"format"=enum."Decimal", "precision"=1}, "visible section"=8} {"minimum" format="%0.2f"; "maximum" format="%0.2f"}
  in  "polar attributes Marker":T10={"maximum"=0.028203326380915113, "minimum"=0.0, "clip to min"=FALSE, "log?(F)"=FALSE, "grid color"=14145495, "plot color"=0, "fmt and prec"={"format"=enum."Decimal", "precision"=1}, "visible section"=8} {"minimum" format="%0.2f"; "maximum" format="%0.2f"}
  in  "polar attributes Prediction":T10={"maximum"=0.0, "minimum"=0.0, "clip to min"=FALSE, "log?(F)"=FALSE, "grid color"=14145495, "plot color"=6618880, "fmt and prec"={"format"=enum."Decimal", "precision"=1}, "visible section"=8} {"minimum" format="%0.2f"; "maximum" format="%0.2f"}
  out "Marker Mag":sgl[][](array[numeric])
